vi "PH_Stepmotor_BaseClass.constructor.vi"(0 "name":string, 2 "data in":string, 5 "error in":errorcluster) -> (14 "i ref out":refnum<vi>, 16 "data out":string, 19 "error out":errorcluster)   [LabVIEW 2014, in "PH_Stepmotor_BaseClass.lvlib"]
doc: "six-pack controller for Trinamics stepper motor controller\n\nauthor: Max Kugler and Stefan Götte, GSI\n\nLicense Agreement for this software:\n\nCopyright (C)\nGesellschaft für Schwerionenforschung, GSI\nPlanckstr. 1\n64291 Darmstadt\nGermany\n\nContact: D.Beck@gsi.de \n\nThis program is free software; you can redistribute it and/or modify it under the terms of the \nGNU General Public License as published by the Free Software Foundation; either version 2 of \nthe license, or (at your option) any later version.\n\nThis program is distributed in the hope that it will be useful, but WITHOUT ANY WARRANTY; \nwithout even the implied warranty of MERCHANTABILITY or FITNESS FOR A PARTICULAR PURPOSE. See the GNU General License for more details (http://www.gnu.org).\n\nGesellschaft für Schwerionenforschung, GSI\nPlanckstr. 1, 64291 Darmstadt, Germany\nFor all questions and ideas contact: M.Richter@gsi.de, H.Brand@gsi.de or D.Beck@gsi.de.\nLast update: 16-JUN-2004"
uses:
  PH_Stepmotor_BaseClass.lvlib
  PH_PSDBWriter/PH_PSDBWriter.Thread Commands.ctl
  PH_PSDBWriter/PH_PSDBWriter.lvlib
  CS_Core/CSSystem/CSSystemLib/CSSystemLib.lvlib
  PH_Class/PH_Class.lvlib
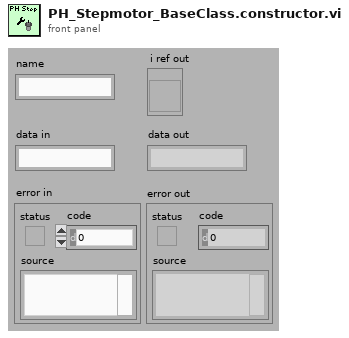
[diagram p1: front panel]
types:
  T1 = enum16{"SetAttribute", "GetAttribute", "CreateAttribute", "DestroyAttribute", "DestroyAllAtributes"}
  T2 = typedef "PH_PSDBWriter.lvlib/PH_PSDBWriter.Thread Commands.ctl" = u16
  T3 = typedef "PH_Stepmotor_BaseClass.lvlib/PH_Stepmotor_BaseClass.i attribute.ctl" = cluster{"Device Error":errorcluster, "Axes PSDB Thread":cluster{"Ref":refnum<vi>, "Q-Ref":refnum<queue>, "Data Status":T4}, "Axes":T5[], "Axes PSDB Infos":cluster{"GUI Name":string, "PSDB Instance ID":i32, "PSDB Status Service ID":i32, "Axis":i32, "Class":string}[], "GUI Refs":T10}
  T4 = typedef "PH_PSDBWriter.lvlib/PH_PSDBWriter.Data Status.ctl" = i16
  T5 = typedef "PH_Stepmotor_BaseClass.lvlib/PH_Stepmotor_BaseClass.Axis Attributes.ctl" = cluster{"Settings":T6, "Endswitch?":bool, "DIM Service IDs":T8, "Activity":T9, "Configured?":bool, "Position":cluster{"Current":i32, "Target":i32}, "Position to set":cluster{"New?":bool, "Wanted":i32}, "Stop?":bool, "Reset?":bool, "Move?":bool, "Nothing connected?":bool}
  T6 = typedef "PH_Stepmotor_BaseClass.lvlib/PH_Stepmotor_BaseClass.Axis Settings.ctl" = cluster{"Sign change":bool, "Width":dbl, "Calibration":dbl, "Unit":string, "Motor Type":T7, "Unit Width":string, "Unit CF":string}
  T7 = typedef "PH_Stepmotor_BaseClass.lvlib/PH_Stepmotor_BaseClass.Motor Type.ctl" = enum16{"Unspecific", "OWIS 49.120.2633", "OWIS 49.060.1033", "OWIS 43.040.2558", "Diamond Motion 2200 series", "OWIS 49.120.266B.MV6", "Calorimeter", "Linear Stage 1", "MICOS VT-80", "MICOS VT-80 S", "Standa Rotstage nt0.95A", "PUF RA 320.200", "PUF RA 800.200", "PUF RA 800.400", "PUF RA 400.50", "1324.nn.800.50", "1324.n9c.800.50", "1324.nn.320.200", "1324.nn.400.200", "1324.nn.800.200", "1324.nn.400.50", "1324.8c9c.800.50", "1324.8c9c.400.200"}
  T8 = typedef "PH_Stepmotor_BaseClass.lvlib/PH_Stepmotor_BaseClass.Axis DIM Service IDs.ctl" = cluster{"Settings":i32, "Information":i32}
  T9 = typedef "PH_Stepmotor_BaseClass.lvlib/PH_Stepmotor_BaseClass.Axis Activity.ctl" = enum16{"No Information", "stopped", "running", "Failure", "Alarm", "stopped at backward ES", "stopped at foreward ES"}
  T10 = typedef "PH_Stepmotor_BaseClass.lvlib/PH_Stepmotor_BaseClass.GUI Refs.ctl" = cluster{"Axes Configuration":refnum<vi>, "Device Error":refnum<vi>, "Axes PSDB Infos":refnum<vi>}
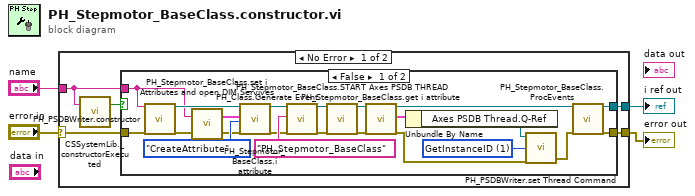
[diagram p0: block diagram]
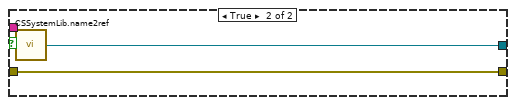
[diagram p2: hidden frame]
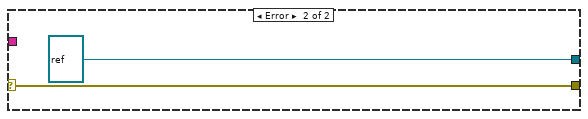
[diagram p3: hidden frame]
diagram:
  n1 = case shown="No Error" "error in" {
    selector: "error in" -> [w9 w36]
    tunnel: "name" -> [w6 _]
    tunnel: [w7 refnum<vi> refnum ("i ref out")] -> w3
    tunnel: [w8 w36] -> w2
    frame No Error {
      n2 = call "CSSystemLib._constructorExecuted.vi"("name"=w6) -> ("constructor executed?"=w5:bool)  [unwired: 18 in]
      n3 = case shown="False" w5 {
        tunnel: w9 -> [w13 w32]
        tunnel: [w30 w32] -> w8
        tunnel: [w29 w33] -> w7
        tunnel: w6 -> [w10 w34]
        frame False {
          w22 = T2 1 items=["None", "GetInstanceID", "WriteToPSDB"] ("PSDB Thread Command")
          n4 = call "PH_PSDBWriter.constructor.vi"("name"=w10, "error in"=w13) -> ("i ref out"=w26:refnum<vi>, "error out"=w12:errorcluster)  [unwired: 15 in, 1 out]
          n5 = call "PH_Stepmotor_BaseClass.set i Attributes and open DIM Servives.vi"("error in"=w12, "Instance Name"=w10) -> ("error out"=w11:errorcluster, "i Attribute"=w27:T3)
          n6 = call "PH_Stepmotor_BaseClass.i attribute.vi"("VI Refnum"=w26, "CLASS.i attribute"=w27, "Action"=T1."CreateAttribute", "error in (no error)"=w11) -> ("VI Refnum out"=w14:refnum<vi>, "error out"=w17:errorcluster)  [unwired: 13 in, 1 out]
          n7 = call "PH_Class.Generate Event.vi"("i ref in"=w14, "Class"="PH_Stepmotor_BaseClass", "error in (no error)"=w17) -> ("i ref out"=w15:refnum<vi>, "error out"=w16:errorcluster)  [unwired: 15 in]
          n8 = call "PH_Stepmotor_BaseClass.START Axes PSDB THREAD.vi"("VI in"=w15, "error in (no error)"=w16) -> ("VI out"=w25:refnum<vi>, "error out"=w20:errorcluster)  [unwired: 16 in]
          n9 = call "PH_Stepmotor_BaseClass.get i attribute.vi"("i ref in"=w25, "error in (no error)"=w20) -> ("i ref out"=w21:refnum<vi>, "i attribute"=w24:T3, "error out"=w19:errorcluster)  [unwired: 15 in]
          n10 = Unbundle By Name(w24) -> ("Axes PSDB Thread.Q-Ref"=w23:refnum<queue>)
          n11 = call "PH_PSDBWriter.set Thread Command.vi"("error in (no error)"=w19, "PSDB Thread Command"=w22, "Queue in"=w23) -> ("error out"=w18:errorcluster)  [unwired: 2 in]
          n12 = call "PH_Stepmotor_BaseClass.ProcEvents.vi"("i ref in"=w21, "error in"=w18) -> ("i ref out"=w29:refnum<vi>, "error out"=w30:errorcluster)  [unwired: 16 in]
        }
        frame True {
          n13 = call "CSSystemLib.name2ref.vi"("name"=w34) -> ("obj refnum"=w33:refnum<vi>)
        }
      }
    }
    frame Error {
    }
  }
  "i ref out" <- w3
  "error out" <- w2
